vi "Create.vi"(9 "Alias":string, 10 "Actor":refnum<class "Actor.lvclass">, 11 "Create in":refnum<class "Create.lvclass">) -> (0 "error out":errorcluster, 3 "Create out":refnum<class "Create.lvclass">)   [LabVIEW 2021, in "Create.lvlib" / "Create.lvclass"]
uses:
  Create.lvclass
  AAM/Actor/Actor.lvclass
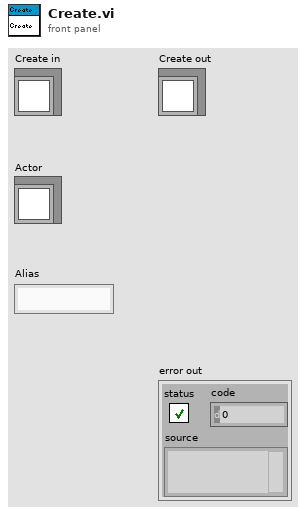
[diagram p1: front panel]
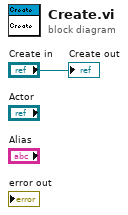
[diagram p0: block diagram]
diagram:
  "Create out" <- "Create in"
